vi "Edit Connector Pane for Wrapper Indicators.vi"(0 "con pane in":refnum<vi>, 5 "indicators in[]":refnum<vi>[](array[refnum]), 11 "error in":errorcluster) -> (4 "con pane out":refnum<vi>, 15 "error out":errorcluster)   [LabVIEW 2021, in "Converter.lvlib"]
uses:
  Converter.lvlib
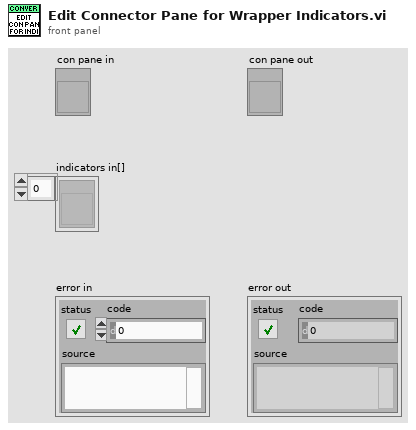
[diagram p1: front panel]
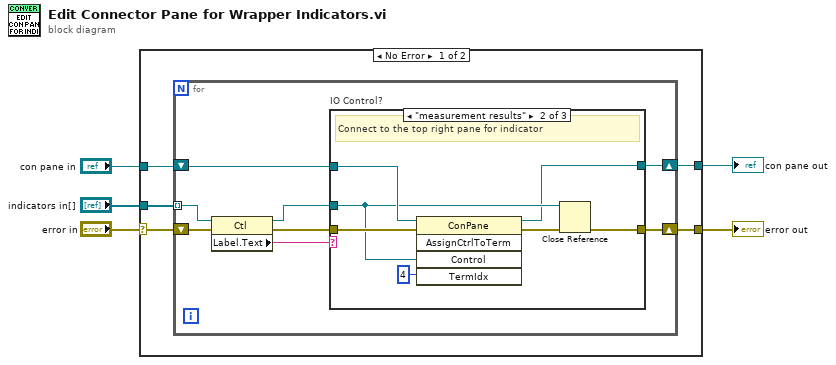
[diagram p0: block diagram]
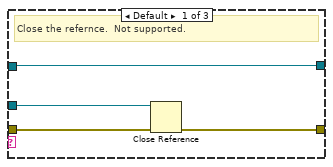
[diagram p2: hidden frame]
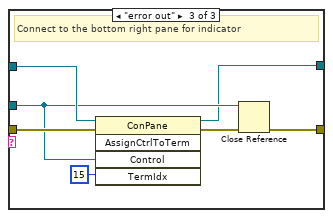
[diagram p3: hidden frame]
diagram:
  n1 = case shown="No Error" "error in" {
    selector: "error in" -> [w8 w37]
    tunnel: "indicators in[]" -> [w10 _]
    tunnel: "con pane in" -> [w9 w38]
    tunnel: [w7 w37] -> w2
    tunnel: [w6 w38] -> w1
    frame No Error {
      n2 = for {
        tunnel: w10 -> [w18] mode=indexing
        shift-right: [w14] -> w7
        shift-left: w8 -> [w13]
        shift-right: [w11] -> w6
        shift-left: w9 -> [w16]
        n3 = property class="Ctl"(reference=w18, error in=w13) -> (reference out=w15:refnum<vi>, error out=w17:errorcluster, "Label.Text"=w12:string)
        n4 = case "IO Control?" shown="\"measurement results\"" w12 {
          tunnel: w17 -> [w22 w26 w33]
          tunnel: w16 -> [w19 w28 w35]
          tunnel: w15 -> [w20 w25 w32]
          tunnel: [w21 w29 w36] -> w14
          tunnel: [w19 w23 w30] -> w11
          frame Default {
            # "Close the refernce.  Not supported."
            n5 = Close Reference(reference=w20, error in (no error)=w22) -> (error out=w21:errorcluster)
          }
          frame "measurement results" {
            # "Connect to the top right pane for indicator"
            n6 = invoke class="ConPane" method="AssignCtrlToTerm"(reference=w28, error in=w26, "Control"=w25, "TermIdx"=u32 4 ("Terminal Index")) -> (reference out=w23:refnum<vi>, error out=w27:errorcluster)  [unwired: 1 in, 3 out]
            n7 = Close Reference(reference=w25, error in (no error)=w27) -> (error out=w29:errorcluster)
          }
          frame "error out" {
            # "Connect to the bottom right pane for indicator"
            n8 = invoke class="ConPane" method="AssignCtrlToTerm"(reference=w35, error in=w33, "Control"=w32, "TermIdx"=u32 15 ("Terminal Index")) -> (reference out=w30:refnum<vi>, error out=w34:errorcluster)  [unwired: 1 in, 3 out]
            n9 = Close Reference(reference=w32, error in (no error)=w34) -> (error out=w36:errorcluster)
          }
        }
      }
    }
    frame Error {
    }
  }
  "error out" <- w2
  "con pane out" <- w1
